vi "IsBlockedCode.vi"(7 "SnakesOnly?":bool, 10 "Code":u32, 11 "SnakeGame in":refnum<class "SnakeGame.lvclass">) -> (2 "Blocked?":bool, 3 "SnakeGame out":refnum<class "SnakeGame.lvclass">)   [LabVIEW 2019, in "RT_Game.lvlib" / "SnakeGame.lvclass"]
uses:
  SnakeGame.lvclass
  SnakeGame.lvclass/SnakeGame.ctl
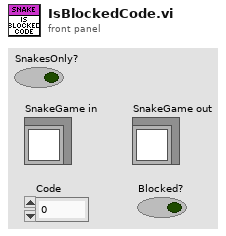
[diagram p1: front panel]
types:
  T1 = cluster{"Head":u32, "Horizontal":u32, "Vertical":u32, "upLeft":u32, "upRight":u32, "downLeft":u32, "downRight":u32}
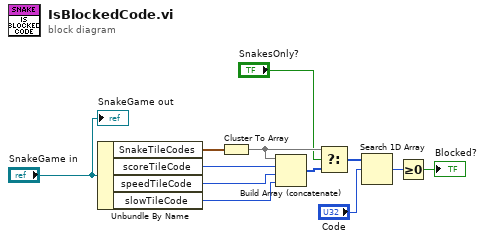
[diagram p0: block diagram]
diagram:
  n1 = Unbundle By Name("SnakeGame in") -> ("SnakeTileCodes"=w11:T1, "scoreTileCode"=w6:u32, "speedTileCode"=w5:u32, "slowTileCode"=w4:u32)
  n2 = Cluster To Array(cluster=w11) -> (array=w2:u32[])
  n3 = Build Array (concatenate)(w2, w6, w5, w4) -> (w7:u32[])
  n4 = Select(t=w2, s="SnakesOnly?", f=w7) -> (s? t:f=w3:u32[])
  n5 = Search 1D Array(1D array=w3, element="Code") -> (index of element=w9:i32)  [unwired: 1 in]
  n6 = Greater Or Equal To 0?(x=w9) -> (x >= 0?=→"Blocked?":bool)
  "SnakeGame out" <- "SnakeGame in"
